vi "16-Bit Down Counter Controller(David Documentation).vi"(7 "Input":u16, 8 "Decrement":bool, 9 "Load":bool, 11 "Value":u16) -> (3 "Value+":u16)   [LabVIEW 2015]
doc: "16-Bit Counting Down"
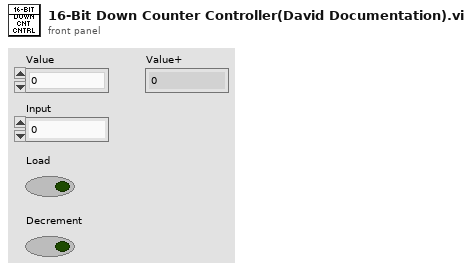
[diagram p1: front panel]
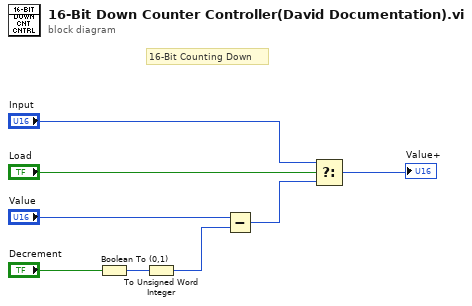
[diagram p0: block diagram]
diagram:
  # "16-Bit Counting Down"
  n1 = Boolean To (0,1)(Boolean="Decrement") -> (0, 1=w4:i16)
  n2 = To Unsigned Word Integer(number=w4) -> (unsigned 16bit integer=w3:u16)
  n3 = Subtract(x="Value", y=w3) -> (x-y=w2:u16)
  n4 = Select(t="Input", s="Load", f=w2) -> (s? t:f=→"Value+":u16)
